vi "Configure pulse amplitude and polarisation.vi"(6 "channel":i32=1 min=1 max=4, 8 "error in (no error)":errorcluster, 9 "offset (0V)":dbl min=0.005 max=5.0, 10 "amplitude (0.01 V)":dbl=0.01 min=0.01 max=5.0, 11 "VISA resource name":refnum<visa-resource-name>="PG-AT") -> (0 "error out":errorcluster, 3 "VISA resource name out":refnum<visa-resource-name>="PG-AT")   [LabVIEW 2019, in "Pulse Rider PG-1000.lvlib"]
uses:
  <instrlib>/Pulse Rider PG-1000/Pulse Rider PG-1000.lvlib
  <instrlib>/Pulse Rider PG-1000/Public/Configure/Pulse/Polarity.ctl
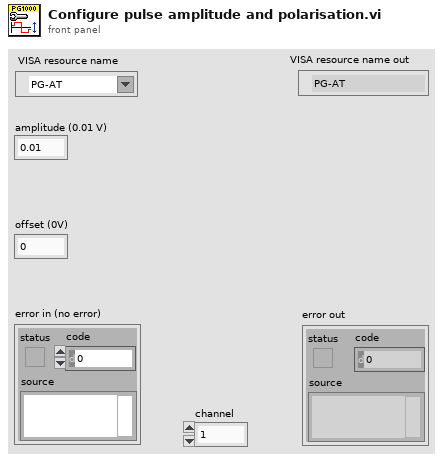
[diagram p1: front panel]
types:
  T1 = typedef "Pulse Rider PG-1000.lvlib/Polarity.ctl" = u16
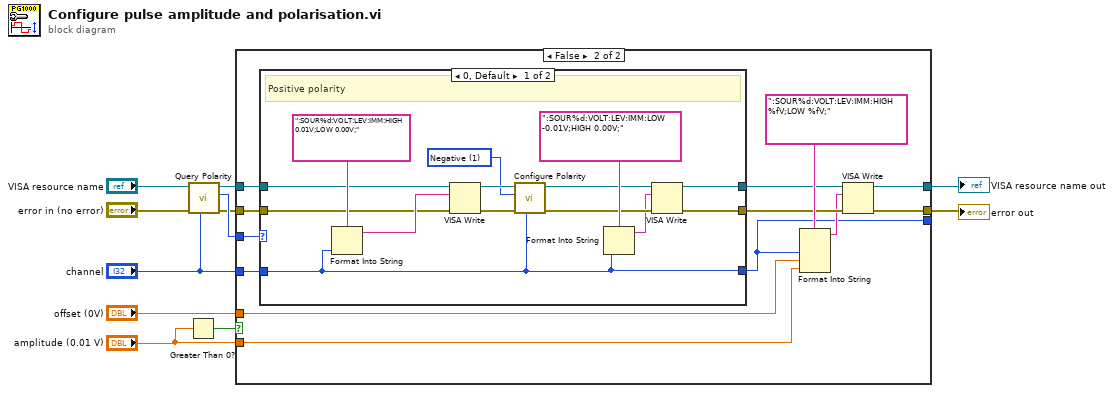
[diagram p0: block diagram]
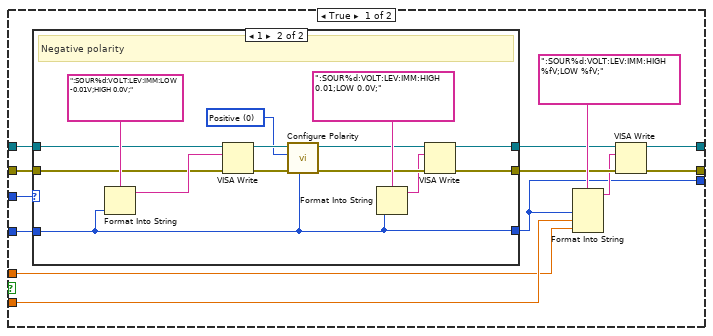
[diagram p2: hidden frame]
diagram:
  n1 = Greater Than 0?(x="amplitude (0.01 V)") -> (x > 0?=w11:bool)
  n2 = call <instrlib>:"Query Polarity.vi"("channel"="channel", "error in (no error)"="error in (no error)", "VISA resource name"="VISA resource name") -> ("error out"=w6:errorcluster, "polarity"=w9:T1, "VISA resource name out"=w7:refnum<visa-resource-name>)  [unwired: 6 in]
  n3 = case shown="False" w11 {
    tunnel: w9 -> [w24 w54]
    tunnel: "channel" -> [w23 w53]
    tunnel: w7 -> [w22 w52]
    tunnel: w6 -> [w21 w51]
    tunnel: "amplitude (0.01 V)" -> [w16 w43]
    tunnel: [w15 w46] -> w3
    tunnel: [w14 w45] -> w2
    tunnel: "offset (0V)" -> [w13 w44]
    tunnel: [w12 w42] -> _
    frame True {
      n4 = case shown="1" w24 {
        tunnel: w23 -> [w25 w28]
        tunnel: w22 -> [w27 w39]
        tunnel: w21 -> [w26 w38]
        tunnel: [w27 w30] -> w19
        tunnel: [w26 w29] -> w18
        tunnel: [w25 w28] -> w12
        frame 0, Default {
          # "Positive polarity"
        }
        frame 1 {
          w35 = T1 0 items=["Positive", "Negative"] ("Polarity (0: Positive)")
          # "Negative polarity"
          n5 = Format Into String(format string=":SOUR%d:VOLT:LEV:IMM:LOW -0.01V;HIGH 0.0V;", w28) -> (resulting string=w40:string)  [unwired: 2 in, 1 out]
          n6 = VISA Write(VISA resource name=w39, write buffer=w40, error in (no error)=w38) -> (VISA resource name out=w37:refnum<visa-resource-name>, error out=w36:errorcluster)  [unwired: 1 out]
          n7 = call <instrlib>:"Configure Polarity.vi"("channel (1)"=w28, "error in (no error)"=w36, "Polarity (0: Positive)"=w35, "VISA resource name"=w37) -> ("error out"=w33:errorcluster, "VISA resource name out"=w32:refnum<visa-resource-name>)  [unwired: 6 in]
          n8 = Format Into String(format string=":SOUR%d:VOLT:LEV:IMM:HIGH 0.01;LOW 0.0V;", w28) -> (resulting string=w31:string)  [unwired: 2 in, 1 out]
          n9 = VISA Write(VISA resource name=w32, write buffer=w31, error in (no error)=w33) -> (VISA resource name out=w30:refnum<visa-resource-name>, error out=w29:errorcluster)  [unwired: 1 out]
        }
      }
      n10 = Format Into String(format string=":SOUR%d:VOLT:LEV:IMM:HIGH %fV;LOW %fV;", w12, w16, w13) -> (resulting string=w17:string)  [unwired: 2 in, 1 out]
      n11 = VISA Write(VISA resource name=w19, write buffer=w17, error in (no error)=w18) -> (VISA resource name out=w15:refnum<visa-resource-name>, error out=w14:errorcluster)  [unwired: 1 out]
    }
    frame False {
      n12 = case shown="0, Default" w54 {
        tunnel: w53 -> [w55 w69]
        tunnel: w52 -> [w66 w71]
        tunnel: w51 -> [w65 w70]
        tunnel: [w57 w71] -> w49
        tunnel: [w56 w70] -> w48
        tunnel: [w55 w69] -> w42
        frame 0, Default {
          w62 = T1 1 items=["Positive", "Negative"] ("Polarity (0: Positive)")
          # "Positive polarity"
          n13 = Format Into String(format string=":SOUR%d:VOLT:LEV:IMM:HIGH 0.01V;LOW 0.00V;", w55) -> (resulting string=w67:string)  [unwired: 2 in, 1 out]
          n14 = VISA Write(VISA resource name=w66, write buffer=w67, error in (no error)=w65) -> (VISA resource name out=w64:refnum<visa-resource-name>, error out=w63:errorcluster)  [unwired: 1 out]
          n15 = call <instrlib>:"Configure Polarity.vi"("channel (1)"=w55, "error in (no error)"=w63, "Polarity (0: Positive)"=w62, "VISA resource name"=w64) -> ("error out"=w60:errorcluster, "VISA resource name out"=w59:refnum<visa-resource-name>)  [unwired: 6 in]
          n16 = Format Into String(format string=":SOUR%d:VOLT:LEV:IMM:LOW -0.01V;HIGH 0.00V;", w55) -> (resulting string=w58:string)  [unwired: 2 in, 1 out]
          n17 = VISA Write(VISA resource name=w59, write buffer=w58, error in (no error)=w60) -> (VISA resource name out=w57:refnum<visa-resource-name>, error out=w56:errorcluster)  [unwired: 1 out]
        }
        frame 1 {
          # "Negative polarity"
        }
      }
      n18 = Format Into String(format string=":SOUR%d:VOLT:LEV:IMM:HIGH %fV;LOW %fV;", w42, w44, w43) -> (resulting string=w47:string)  [unwired: 2 in, 1 out]
      n19 = VISA Write(VISA resource name=w49, write buffer=w47, error in (no error)=w48) -> (VISA resource name out=w46:refnum<visa-resource-name>, error out=w45:errorcluster)  [unwired: 1 out]
    }
  }
  "VISA resource name out" <- w3
  "error out" <- w2
